vi "pythjTheorem.vi"(10 "yDistance":dbl, 11 "xDistance":dbl) -> (3 "autoDistance":dbl)   [LabVIEW 2017]
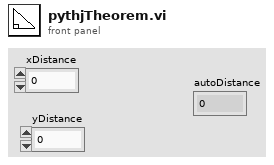
[diagram p1: front panel]
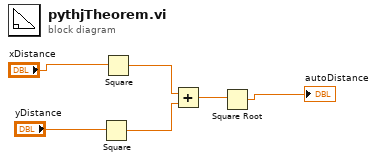
[diagram p0: block diagram]
diagram:
  n1 = Square(x="yDistance") -> (x^2=w3:dbl)
  n2 = Square(x="xDistance") -> (x^2=w4:dbl)
  n3 = Add(x=w4, y=w3) -> (x+y=w2:dbl)
  n4 = Square Root(x=w2) -> (sqrt(x)=→"autoDistance":dbl)
